vi "UpdateControlsFromSettingsFile.vi"(9 "name or relative path":string="Robomos", 10 "Array":refnum<vi>[](array[refnum]), 11 "Path in":refnum<vi>) -> (3 "dup path":path)   [LabVIEW 2015]
uses:
  <vilib>/Utility/sysdir.llb/System Directory Type.ctl
  <vilib>/Utility/file.llb/Read Delimited Spreadsheet (string).vi
panel:
  out "error out":errorcluster
  in  "error in (no error)":errorcluster
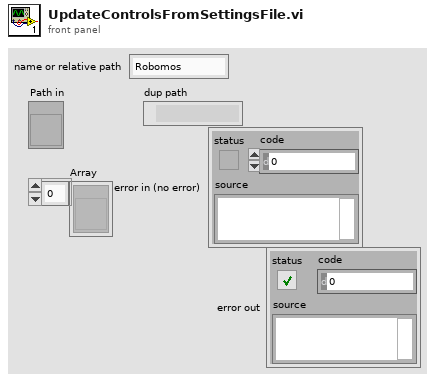
[diagram p1: front panel]
types:
  T1 = typedef "System Directory Type.ctl" = i32
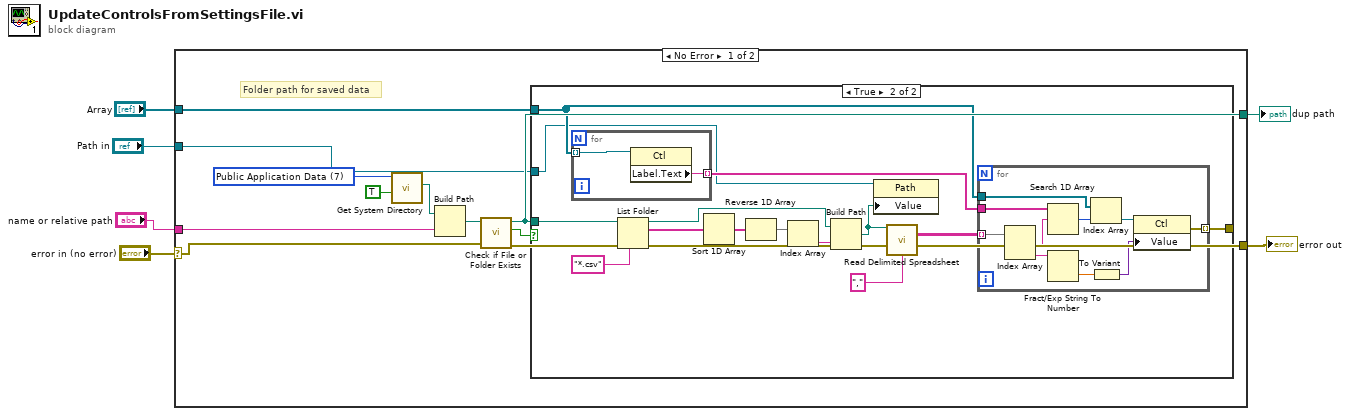
[diagram p0: block diagram]
diagram:
  n1 = case shown="No Error" "error in (no error)" {
    selector: "error in (no error)" -> [w9 w44]
    tunnel: "Array" -> [w17 _]
    tunnel: [w16 _] -> w5
    tunnel: "Path in" -> [w10 _]
    tunnel: [w8 w44] -> w2
    tunnel: "name or relative path" -> [w7 _]
    frame No Error {
      w12 = T1 7 items=["User Home"=0, "User Desktop"=1, "User Documents"=2, "User Application Data"=3, "User Preferences"=4, "User Temporary"=5, "Public Documents"=6, "Public Application Data"=7, "Public Preferences"=8, "Public Cache"=13, "System Core Libraries"=9, "System Installed Libraries"=10, "Application Files"=11, "Boot Volume Root"=12] ("system directory type")
      # "Folder path for saved data"
      n2 = call <vilib>:"Get System Directory.vi"("create directory if not found? (F)"=TRUE, "system directory type"=w12) -> ("system directory"=w13:path)  [unwired: 9 in]
      n3 = Build Path(base path=w13, name or relative path=w7) -> (appended path=w11:path)
      n4 = call <vilib>:"Check if File or Folder Exists.vi"("error in (no error)"=w9, "path"=w11) -> ("error out"=w8:errorcluster, "file or folder exists?"=w15:bool, "dup path"=w16:path)  [unwired: 7 in]
      n5 = case shown="True" w15 {
        tunnel: w16 -> [_ w31]
        tunnel: w17 -> [_ w23]
        tunnel: [_ w22] -> _
        tunnel: w10 -> [_ w21]
        frame False {
        }
        frame True {
          n6 = for {
            tunnel: w23 -> [w33] mode=indexing
            tunnel: [w32] -> w24 mode=indexing
            n7 = property class="Ctl"(reference=w33) -> ("Label.Text"=w32:string)  [unwired: 1 in, 2 out]
          }
          n8 = List Folder(path=w31, pattern="*.csv") -> (path out=w25:path, filenames=w29:string[])  [unwired: 2 in, 2 out]
          n9 = Sort 1D Array(array=w29) -> (sorted array=w28:string[])
          n10 = Reverse 1D Array(array=w28) -> (reversed array=w27:string[])
          n11 = Index Array(array=w27) -> (element=w26:string)  [unwired: 1 in]
          n12 = Build Path(base path=w25, name or relative path=w26) -> (appended path=w20:path)
          n13 = property class="Path"(reference=w21, "Value"=w20) -> ()  [unwired: 1 in, 2 out]
          n14 = call-poly <vilib>:"Read Delimited Spreadsheet.vi"("file path (dialog if empty)"=w20, "delimiter (\\t)"="," ("delimiter (\\t)")) -> ("all rows"=w18:string[][])  [unwired: 8 in, 5 out]
          n15 = for {
            tunnel: w18 -> [w43] mode=indexing
            tunnel: w24 -> [w42]
            tunnel: w23 -> [w40]
            tunnel: [w37] -> w22 mode=indexing
            n16 = Index Array(array=w43) -> (element #1=w41:string, element #2=w39:string)  [unwired: 2 in]
            n17 = Search 1D Array(1D array=w42, element=w41) -> (index of element=w38:i32)  [unwired: 1 in]
            n18 = Fract/Exp String To Number(string=w39) -> (number=w35:dbl)  [unwired: 3 in, 1 out]
            n19 = Index Array(array=w40, index=w38) -> (element=w36:refnum<vi>)
            n20 = To Variant(anything=w35) -> (Variant=w34:variant)
            n21 = property class="Ctl"(reference=w36, "Value"=w34) -> (error out=w37:errorcluster)  [unwired: 1 in, 1 out]
          }
        }
      }
    }
    frame Error {
    }
  }
  "dup path" <- w5
  "error out" <- w2
